vi "Code Hexadecimal 16 Relais.vi"(8 "Error In":errorcluster caption="Entrée d'erreur", 9 "Etat":bool, 10 "référence":refnum<vi>, 11 "tableau code":u8[](array[numeric]) format="%x") -> (0 "Error Out":errorcluster caption="Sortie d'erreur", 2 "référence en sortie":refnum<vi>, 3 "tableau en sortie":u8[](array[numeric]) format="%x")   [LabVIEW 2017]
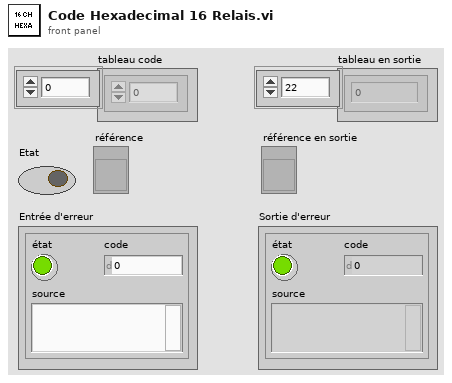
[diagram p1: front panel]
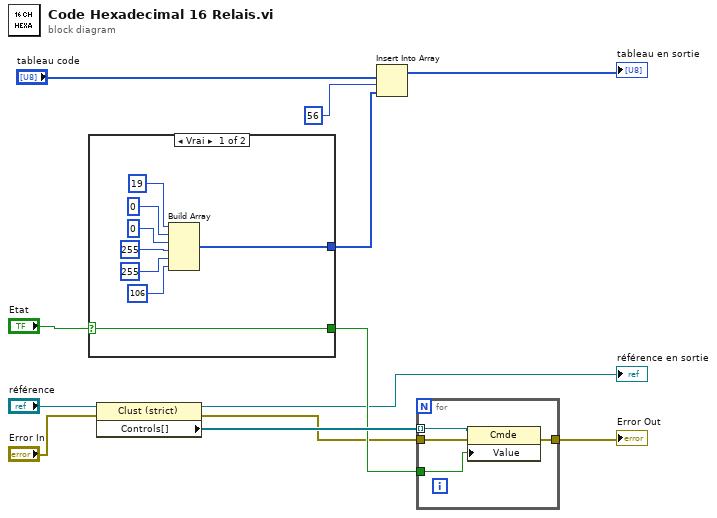
[diagram p0: block diagram]
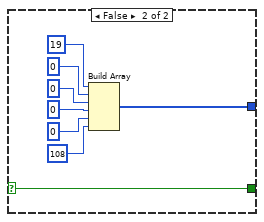
[diagram p2: hidden frame]
diagram:
  n1 = case shown="Vrai" "Etat" {
    selector: "Etat" -> [w13 w21]
    tunnel: [w14 w22] -> w8
    tunnel: [w13 w21] -> w6
    frame True {
      n2 = Build Array(u8 19 ("élément"), u8 0 ("élément"), u8 0 ("élément"), u8 255 ("élément"), u8 255 ("élément"), u8 106 ("élément")) -> (w14:u8[])
    }
    frame False {
      n3 = Build Array(u8 19 ("élément"), u8 0 ("élément"), u8 0 ("élément"), u8 0 ("élément"), u8 0 ("élément"), u8 108 ("élément")) -> (w22:u8[])
    }
  }
  n4 = property class="Clust (strict)"(reference="référence", error in="Error In") -> (reference out=→"référence en sortie":refnum<vi>, error out=w1:errorcluster, "Controls[]"=w7:refnum<vi>[])
  n5 = Insert Into Array(array="tableau code", index=56 ("indice"), new element=w8) -> (→"tableau en sortie":u8[])
  n6 = for {
    tunnel: w7 -> [w32] mode=indexing
    tunnel: w6 -> [w31]
    tunnel: [w30] -> w4
    tunnel: w1 -> [w29]
    n7 = property class="Cmde"(reference=w32, error in=w29, "Value"=w31) -> (error out=w30:errorcluster)  [unwired: 1 out]
  }
  "Error Out" <- w4
